vi "Write Blob to PAS Board.vi"(0 "Session Handle in":T1, 1 "Reverse?":bool, 5 "Bytes to Write":u8[](array[numeric]), 11 "error in (no error)":errorcluster) -> (4 "Session Handle out":T1, 15 "error out":errorcluster)   [LabVIEW 2015, in "PAS.lvclass"]
uses:
  PAS.lvclass
  Typedefs/Session Handle.ctl
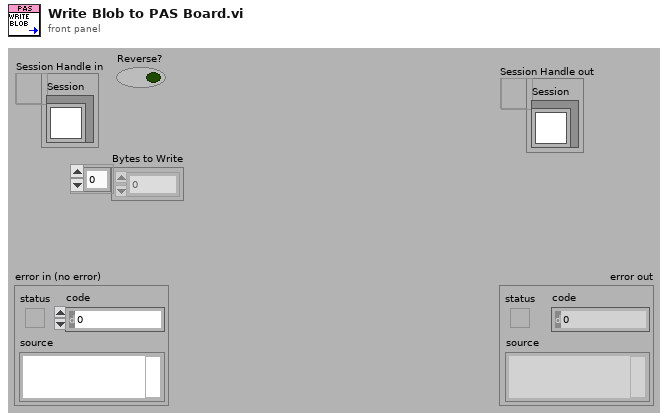
[diagram p1: front panel]
types:
  T1 = typedef "PAS.lvclass/Session Handle.ctl" = refnum<data-value>
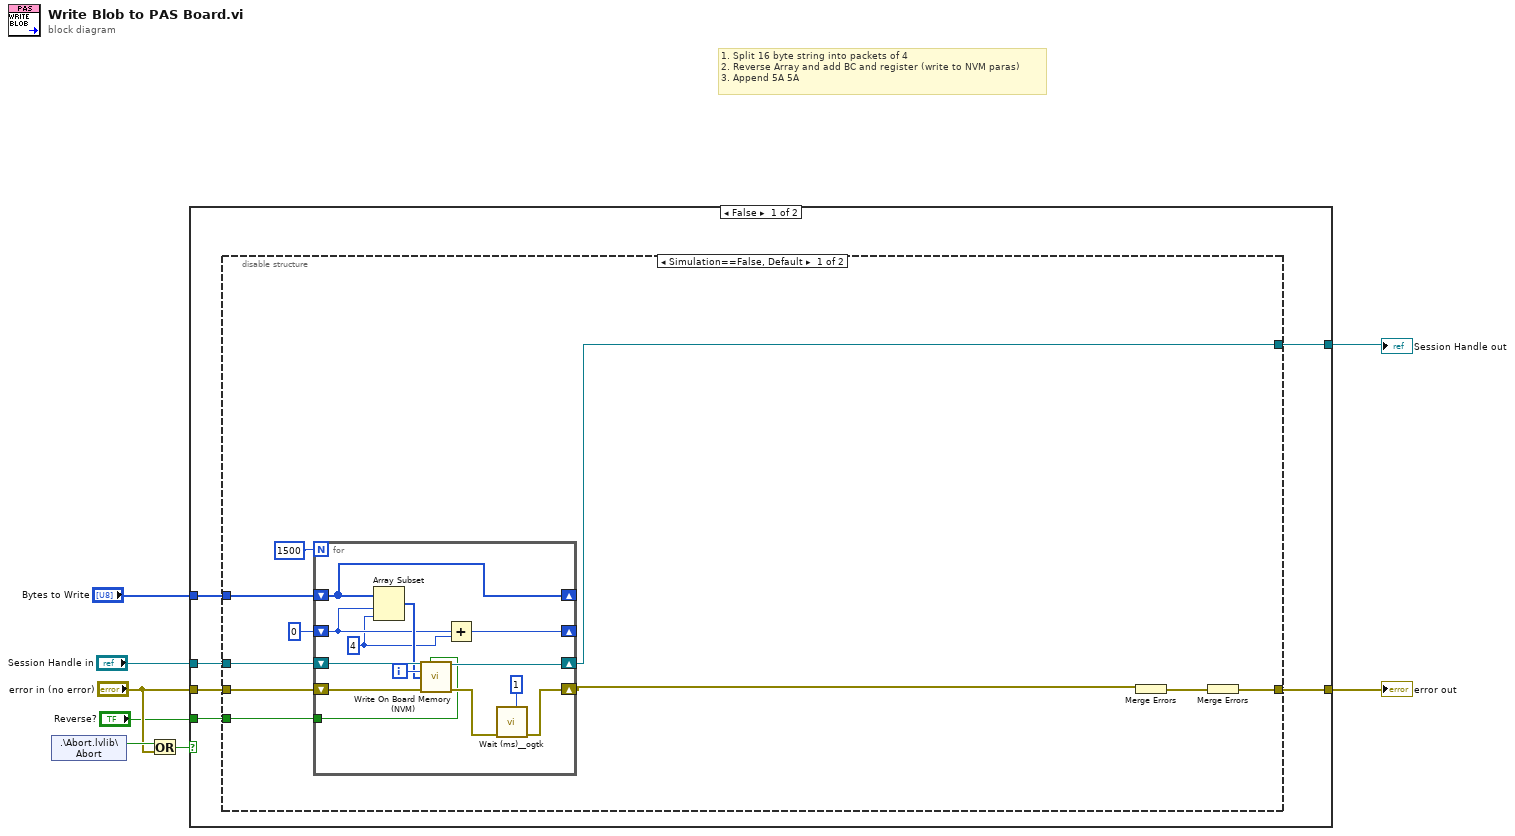
[diagram p0: block diagram]
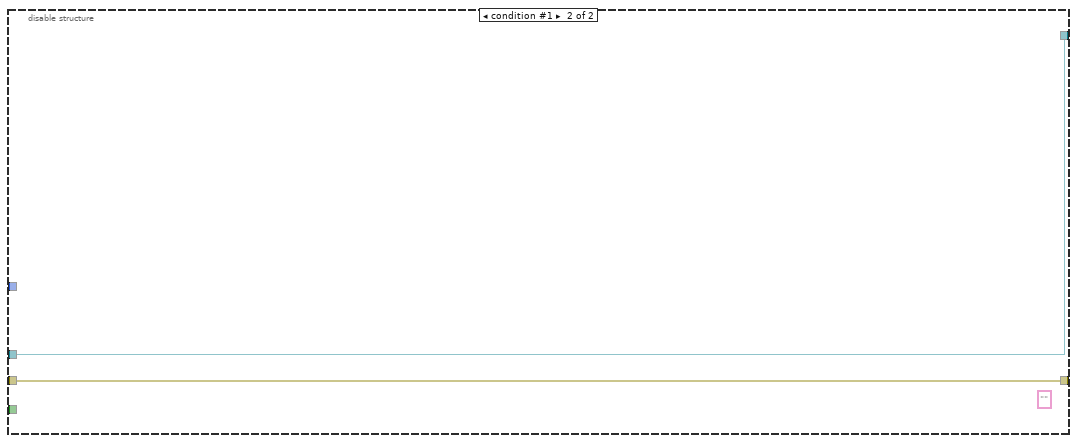
[diagram p2: hidden frame]
diagram:
  # "1. Split 16 byte string into packets of 4\n2. Reverse Array and add BC and register (write to NVM paras)\n3. Append 5A 5A"
  n1 = shared-variable ".\\Abort.lvlib\\Abort"() -> (w5:bool)  [unwired: 1 in, 1 out]
  n2 = Or(x=w5, y="error in (no error)") -> (x .or. y?=w3:bool)
  n3 = case shown="False" w3 {
    tunnel: [w14 w41] -> w7
    tunnel: [w13 w40] -> w6
    tunnel: "Session Handle in" -> [w12 w41]
    tunnel: "error in (no error)" -> [w11 w40]
    tunnel: "Bytes to Write" -> [w10 _]
    tunnel: "Reverse?" -> [w9 _]
    frame False {
      n4 = disable-structure shown="Simulation==False, Default" {
        disable-tunnel: [w16 w39] -> w14
        disable-tunnel: [w23 w38] -> w13
        disable-tunnel: w12 -> [w19 w39]
        disable-tunnel: w11 -> [w22 w38]
        disable-tunnel: w10 -> [w18 _]
        disable-tunnel: w9 -> [w15 _]
        frame condition #0 (active) {
          n5 = for {
            N: 1500 -> [_]
            shift-right: [w27] -> w17
            shift-left: w22 -> [w37]
            shift-right: [w30] -> _
            shift-left: 0 -> [w31]
            shift-right: [w33] -> w16
            shift-left: w19 -> [w36]
            shift-right: [w32] -> _
            shift-left: w18 -> [w32]
            tunnel: w15 -> [w25]
            i -> [w35]
            w29 = 4 ("y")
            n6 = Array Subset(array=w32, index=w31, length=w29) -> (w34:u8[])
            n7 = call "Write On Board Memory (NVM).vi"("Session Handle in"=w36, "Reverse?"=w25, "Address"=w35, "Bytes to Write"=w34, "error in (no error)"=w37) -> ("Session Handle out"=w33:T1, "error out"=w28:errorcluster)  [unwired: 9 in]
            n8 = Add(x=w31, y=w29) -> (x+y=w30:i32)
            n9 = call <userlib>:"Wait (ms)__ogtk.vi"("error in (no error)"=w28, "milliseconds to wait"=u32 1) -> ("error out"=w27:errorcluster)  [unwired: 8 in, 1 out]
          }
          n10 = Merge Errors(w17) -> (w24:errorcluster)
          n11 = Merge Errors(w24) -> (w23:errorcluster)
        }
        frame condition #1 {
          (unwired) "" ("string")
        }
      }
    }
    frame True {
    }
  }
  "Session Handle out" <- w7
  "error out" <- w6
